vi "CPP_DisplayPosAndWait.vi"() -> (5 "Plug in titles":string[](array[string]), 7 "Plug in values":string[](array[string]))   [LabVIEW 2011]
uses:
  Globals/Meas_global.vi
  Globals/Plug_in_data_global.vi
  Globals/ForceWait.vi
  Globals/Trav_pos_global.vi
  Controls/Inst_type.ctl
  Controls/Analysis_info_cluster.ctl
  Controls/Instrument_Array.ctl
  Controls/XY_Plot_Cluster.ctl
panel:
  out "Z":dbl format="%#.0f"
  out "Y":dbl format="%#.0f"
  out "X":dbl format="%#.0f"
  out "Analysis Info cluster":T1[](array[typedef])=[{"Colour"=0, "Inst type"=enum."Pitot-static tube", "Inst name"="Manometer voltage", "Symbol"="U", "Code name"="", "Extra Info"="U", "Inst Array"=enum."PWA", "Index"=0, "Voltage Index"=0, "Extra Titles"=[], "Extra Values"=[], "Eng Values"=[], "Time (ms)"=[], "Voltage"=[], "U"=0.0, "u^2"=0.0, "u^3"=0.0, "u^4"=0.0, "Skew_u"=0.0, "Kurt_u"=0.0, "Sd Error in Mean"=0.0, "% u'/U"=0.0, "X"=0.0, "Y"=0.0, "Z"=0.0, "Spectra"={"First Name"="", "Second Name"="", "X axis name"="", "Y axis name"="", "X array"=[], "Y array"=[]}, "Autocorrelation"={"First Name"="", "Second Name"="", "X axis name"="", "Y axis name"="", "X array"=[], "Y array"=[]}, "Timescale integral to 25%"=0.0, "Sd Error in Variance"=0.0, "Calib File"=path "", "Calib Constants"=[], "Histogram"={"First Name"="", "Second Name"="", "X axis name"="", "Y axis name"="", "X array"=[], "Y array"=[]}, "Output Position"=FALSE, "Full Stats"=FALSE, "Weighting"=[]}, {"Colour"=0, "Inst type"=enum."Pitot-static tube", "Inst name"="Manometer voltage", "Symbol"="U", "Code name"="", "Extra Info"="U", "Inst Array"=enum."PWA", "Index"=0, "Voltage Index"=0, "Extra Titles"=[], "Extra Values"=[], "Eng Values"=[], "Time (ms)"=[], "Voltage"=[], "U"=0.0, "u^2"=0.0, "u^3"=0.0, "u^4"=0.0, "Skew_u"=0.0, "Kurt_u"=0.0, "Sd Error in Mean"=0.0, "% u'/U"=0.0, "X"=0.0, "Y"=0.0, "Z"=0.0, "Spectra"={"First Name"="", "Second Name"="", "X axis name"="", "Y axis name"="", "X array"=[], "Y array"=[]}, "Autocorrelation"={"First Name"="", "Second Name"="", "X axis name"="", "Y axis name"="", "X array"=[], "Y array"=[]}, "Timescale integral to 25%"=0.0, "Sd Error in Variance"=0.0, "Calib File"=path "", "Calib Constants"=[], "Histogram"={"First Name"="", "Second Name"="", "X axis name"="", "Y axis name"="", "X array"=[], "Y array"=[]}, "Output Position"=FALSE, "Full Stats"=FALSE, "Weighting"=[]}, {"Colour"=0, "Inst type"=enum."Pitot-static tube", "Inst name"="Manometer voltage", "Symbol"="U", "Code name"="", "Extra Info"="U", "Inst Array"=enum."PWA", "Index"=0, "Voltage Index"=0, "Extra Titles"=[], "Extra Values"=[], "Eng Values"=[], "Time (ms)"=[], "Voltage"=[], "U"=0.0, "u^2"=0.0, "u^3"=0.0, "u^4"=0.0, "Skew_u"=0.0, "Kurt_u"=0.0, "Sd Error in Mean"=0.0, "% u'/U"=0.0, "X"=0.0, "Y"=0.0, "Z"=0.0, "Spectra"={"First Name"="", "Second Name"="", "X axis name"="", "Y axis name"="", "X array"=[], "Y array"=[]}, "Autocorrelation"={"First Name"="", "Second Name"="", "X axis name"="", "Y axis name"="", "X array"=[], "Y array"=[]}, "Timescale integral to 25%"=0.0, "Sd Error in Variance"=0.0, "Calib File"=path "", "Calib Constants"=[], "Histogram"={"First Name"="", "Second Name"="", "X axis name"="", "Y axis name"="", "X array"=[], "Y array"=[]}, "Output Position"=FALSE, "Full Stats"=FALSE, "Weighting"=[]}, {"Colour"=0, "Inst type"=enum."Pitot-static tube", "Inst name"="Manometer voltage", "Symbol"="U", "Code name"="", "Extra Info"="U", "Inst Array"=enum."PWA", "Index"=0, "Voltage Index"=0, "Extra Titles"=[], "Extra Values"=[], "Eng Values"=[], "Time (ms)"=[], "Voltage"=[], "U"=0.0, "u^2"=0.0, "u^3"=0.0, "u^4"=0.0, "Skew_u"=0.0, "Kurt_u"=0.0, "Sd Error in Mean"=0.0, "% u'/U"=0.0, "X"=0.0, "Y"=0.0, "Z"=0.0, "Spectra"={"First Name"="", "Second Name"="", "X axis name"="", "Y axis name"="", "X array"=[], "Y array"=[]}, "Autocorrelation"={"First Name"="", "Second Name"="", "X axis name"="", "Y axis name"="", "X array"=[], "Y array"=[]}, "Timescale integral to 25%"=0.0, "Sd Error in Variance"=0.0, "Calib File"=path "", "Calib Constants"=[], "Histogram"={"First Name"="", "Second Name"="", "X axis name"="", "Y axis name"="", "X array"=[], "Y array"=[]}, "Output Position"=FALSE, "Full Stats"=FALSE, "Weighting"=[]}] {"Sd Error in Variance" format="%.2f"; "Skew_u" format="%.2f"; "% u'/U" format="%.2f"; "Sd Error in Mean" format="%.2f"; "Kurt_u" format="%.2f"; "u^4" format="%.2f"; "u^3" format="%.2f"; "U" format="%.2f"; "u^2" format="%.2f"}
  out "Current Block No":i32
  out "Raw data file":path
  out "Actual Sampling rate (Hz)":dbl=1000.0 format="%.2f"
  out "Equi Spaced":dbl[][](array[numeric]) format="%.2f"
  # "You must have just these two indicators on the connector pane of the vi"
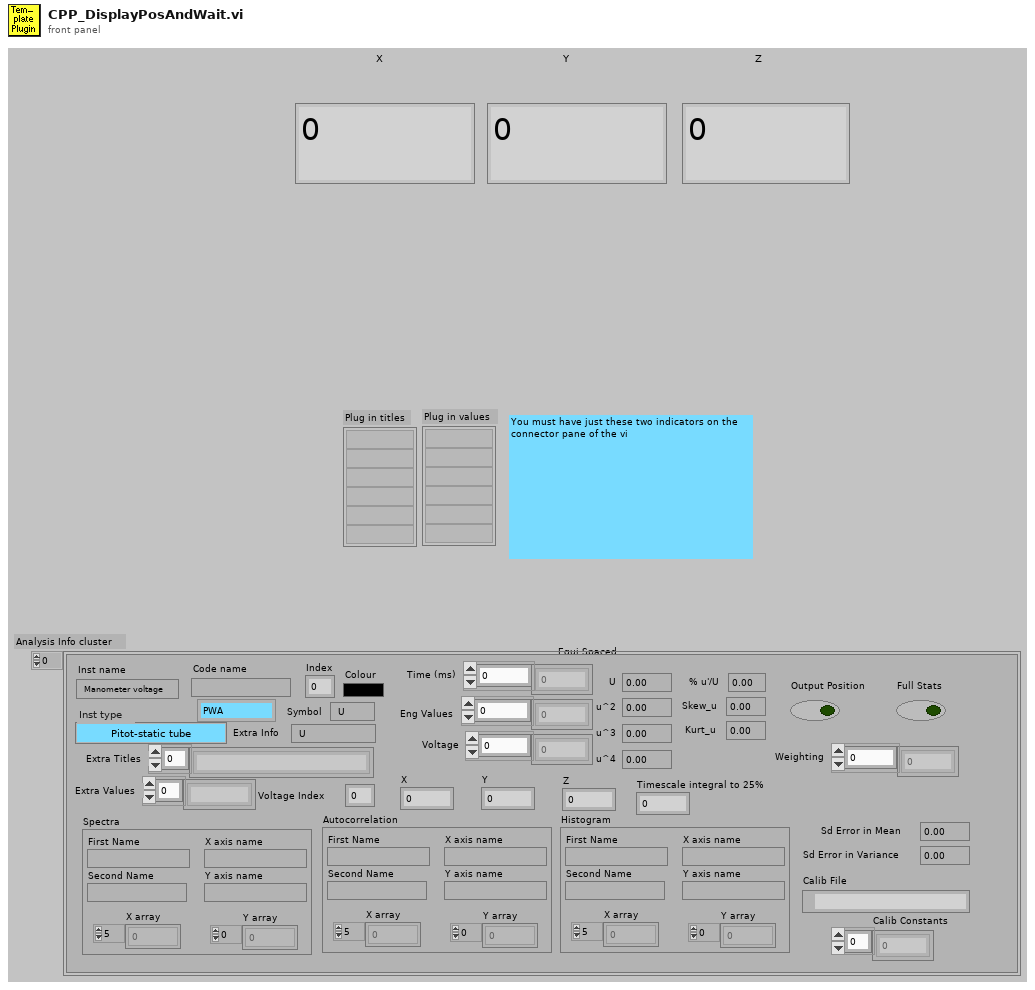
[diagram p1: front panel]
types:
  T1 = typedef "Analysis_info_cluster.ctl" = cluster{"Colour":u32, "Inst type":T2, "Inst name":string, "Symbol":string, "Code name":string, "Extra Info":string, "Inst Array":T3, "Index":i32, "Voltage Index":i32, "Extra Titles":string[], "Extra Values":string[], "Eng Values":dbl[], "Time (ms)":dbl[], "Voltage":dbl[], "U":dbl, "u^2":dbl, "u^3":dbl, "u^4":dbl, "Skew_u":dbl, "Kurt_u":dbl, "Sd Error in Mean":dbl, "% u'/U":dbl, "X":dbl, "Y":dbl, "Z":dbl, "Spectra":T4, "Autocorrelation":T4, "Timescale integral to 25%":dbl, "Sd Error in Variance":dbl, "Calib File":path, "Calib Constants":dbl[], "Histogram":T4, "Output Position":bool, "Full Stats":bool, "Weighting":dbl[]}
  T2 = typedef "Inst_type.ctl" = enum16{"Propeller anemometer", "Raw voltage", "Pressure Transducer", "Pitot-static tube", "Preston tube", "Hot wire", "Cross wire 1", "Cross wire 2", "Generic Linear", "Generic Polynomial", "Generic BackPoly", "Fast FID", "Thermocouple", "Cold wire", "Pulsed Wire", "LDA Vel", "LDA Tran time", "LDA Arr time"}
  T3 = typedef "Instrument_Array.ctl" = enum16{"PWA", "LDA", "Analogue"}
  T4 = typedef "XY_Plot_Cluster.ctl" = cluster{"First Name":string, "Second Name":string, "X axis name":string, "Y axis name":string, "X array":dbl[], "Y array":dbl[]}
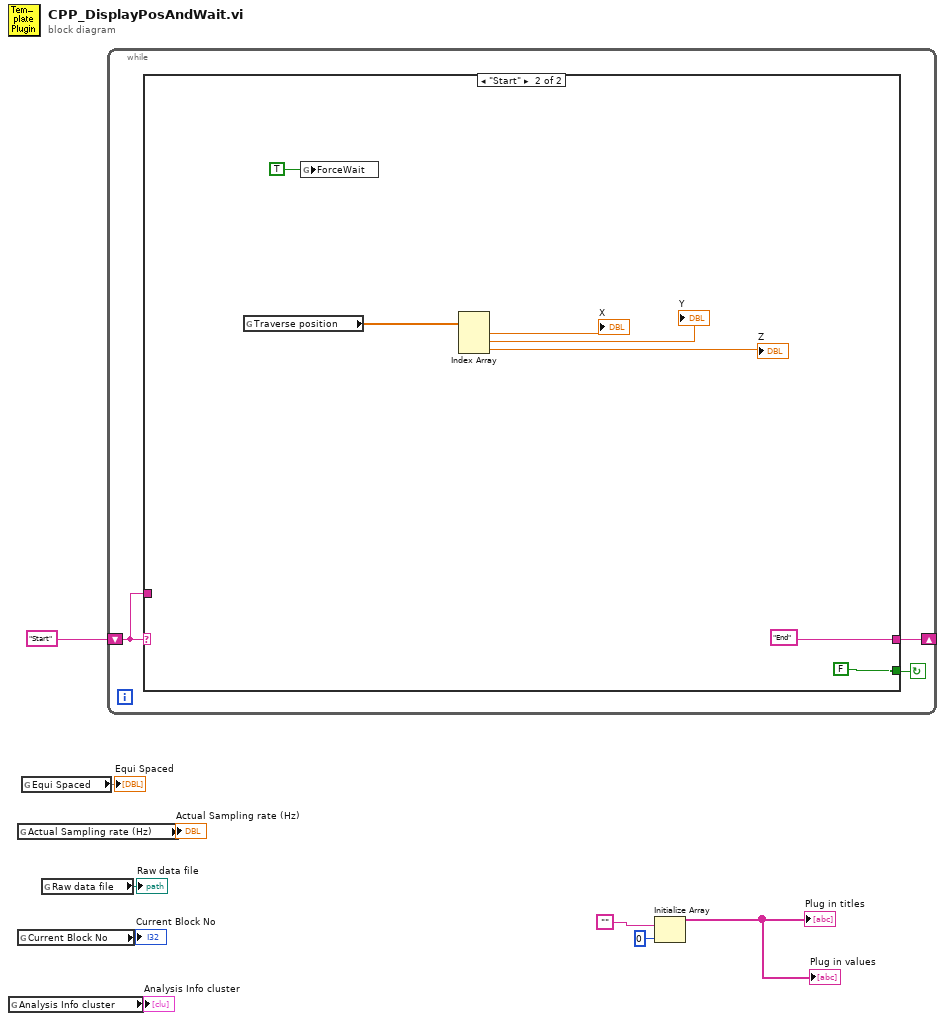
[diagram p0: block diagram]
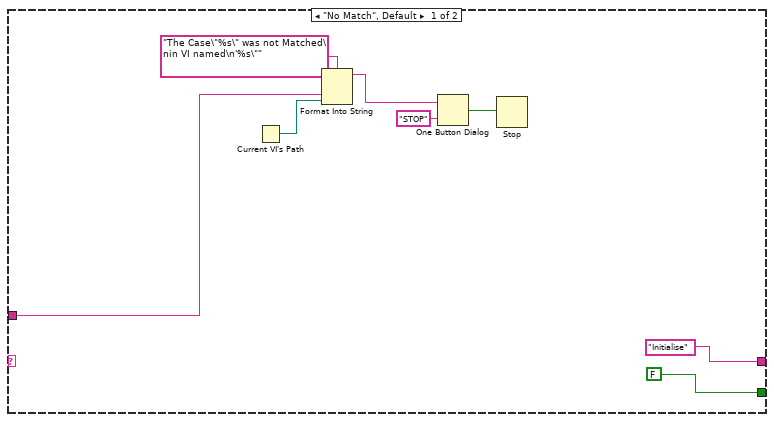
[diagram p2: hidden frame]
diagram:
  n1 = global read "Meas_global.vi" "Analysis Info cluster"() -> (→"Analysis Info cluster":T1[])
  n2 = global read "Meas_global.vi" "Actual Sampling rate (Hz)"() -> (→"Actual Sampling rate (Hz)":dbl)
  n3 = global read "Meas_global.vi" "Current Block No"() -> (→"Current Block No":i32)
  n4 = global read "Plug_in_data_global.vi" "Equi Spaced"() -> (→"Equi Spaced")
  n5 = global read "Meas_global.vi" "Raw data file"() -> (→"Raw data file":path)
  n6 = while {
    shift-left: "Start" -> [w10]
    shift-right: [w11] -> _
    stop <- w12 continue-if-true
    n7 = case shown="\"Start\"" w10 {
      tunnel: [FALSE FALSE] -> w12
      tunnel: ["Initialise" "End"] -> w11
      tunnel: w10 -> [w15 _]
      frame "No Match", Default {
        n8 = Current VI's Path() -> (path=w14:path)
        n9 = Format Into String(format string="The Case\"%s\" was not Matched\nin VI named\n'%s\"" ("Format String"), w15, w14) -> (resulting string=w18:string)  [unwired: 2 in, 1 out]
        n10 = One Button Dialog(message=w18, button name ("OK")="STOP") -> (true=w16:bool)
        n11 = Stop(stop? (T)=w16) -> ()
      }
      frame "Start" {
        n12 = global read "Trav_pos_global.vi" "Traverse position"() -> (w24:dbl[])
        n13 = global write "ForceWait.vi" "ForceWait"(TRUE ("ForceWait")) -> ()
        n14 = Index Array(array=w24) -> (element #1=→"X":dbl, element #2=→"Y":dbl, element #3=→"Z":dbl)  [unwired: 3 in]
      }
    }
  }
  n15 = Initialize Array("", 0) -> (→"Plug in values" →"Plug in titles":string[])
